vi "Luefter ansteuern.vi"(8 "Lüfter schnell":sgl, 9 "Lüfter langsam":sgl, 11 "Schaltschrank":sgl) -> ()   [LabVIEW 2020, in "Allgemein.lvlib"]
uses:
  Allgemein.lvlib
  Regler/FGV Daten Regler Aktionen.ctl
  Regler/Regler.lvlib
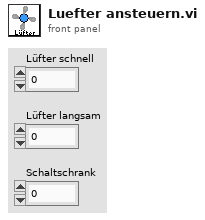
[diagram p1: front panel]
types:
  T1 = typedef "Regler.lvlib/FGV Daten Regler Aktionen.ctl" = enum16{"lesen", "Out%", "Heizung EIN"}
  T2 = cluster{"Output% 1":i16, "Output% 2":i16, "Output% 3":i16, "Output% 4":i16, "Output% 5":i16, "Output% 6":i16, "Output% 7":i16, "Output% 8":i16, "Output% 9":i16, "Output% 10":i16, "Output% 11":i16, "Output% 12":i16, "Output% 13":i16, "Output% 14":i16, "Output% 15":i16, "Output% 16":i16, "Output% 17":i16, "Output% 18":i16}
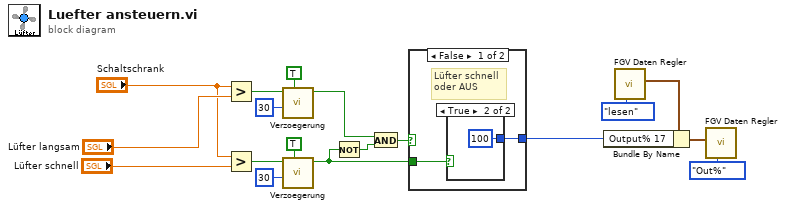
[diagram p0: block diagram]
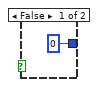
[diagram p2: hidden frame]
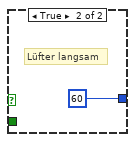
[diagram p3: hidden frame]
diagram:
  n1 = Greater?(x="Schaltschrank", y="Lüfter langsam") -> (0:w4:bool)
  n2 = Greater?(x="Schaltschrank", y="Lüfter schnell") -> (0:w6:bool)
  n3 = call "Verzoegerung.vi"("Abfallverzögerung?"=TRUE, "sec"=u16 30, "Startsignal"=w4) -> ("Zeit abgelaufen?"=w5:bool)  [unwired: 7 in, 1 out]
  n4 = call "Verzoegerung.vi"("Abfallverzögerung?"=TRUE, "sec"=u16 30, "Startsignal"=w6) -> ("Zeit abgelaufen?"=w7:bool)  [unwired: 7 in, 1 out]
  n5 = Not(x=w7) -> (.not. x?=w1:bool)
  n6 = And(x=w5, y=w1) -> (x .and. y?=w2:bool)
  n7 = case shown="False" w2 {
    tunnel: [w20 i16 60 ("Output% 12")] -> w3
    tunnel: w7 -> [w19 _]
    frame False {
      # "Lüfter schnell\noder AUS"
      n8 = case shown="True" w19 {
        tunnel: [i16 0 ("Output% 12") i16 100 ("Output% 12")] -> w20
        frame False {
        }
        frame True {
        }
      }
    }
    frame True {
      # "Lüfter langsam"
    }
  }
  n9 = call "FGV Daten Regler.vi"("Aktionen"=FGV_Daten_Regler_Aktionen."lesen") -> ("PID - OUT%"=w16:T2)  [unwired: 9 in, 1 out]
  n10 = Bundle By Name(cluster=w16, "Output% 17"=w3) -> (w18:T2)
  n11 = call "FGV Daten Regler.vi"("Aktionen"=FGV_Daten_Regler_Aktionen."Out%", "PID - OUT%"=w18) -> ()  [unwired: 8 in, 2 out]
